vi "Log in MsgList.vi"(8 "error in (no error)":errorcluster, 9 "Username (max 15 characters)":string, 10 "Msg":string, 11 "Function in":refnum<class "Function.lvclass">) -> (0 "error out":errorcluster, 3 "Function out":refnum<class "Function.lvclass">)   [LabVIEW 2016, in "Function Actor.lvlib" / "Function.lvclass"]
uses:
  <userlib>/Common Components/Function Actor/Function.lvclass
  <userlib>/Common Components/Function Actor/Function.lvclass/Function.ctl
  <userlib>/Common Components/Common/Msg MCLstBox Append.vi
  <userlib>/Common Components/Common/Common.lvlib
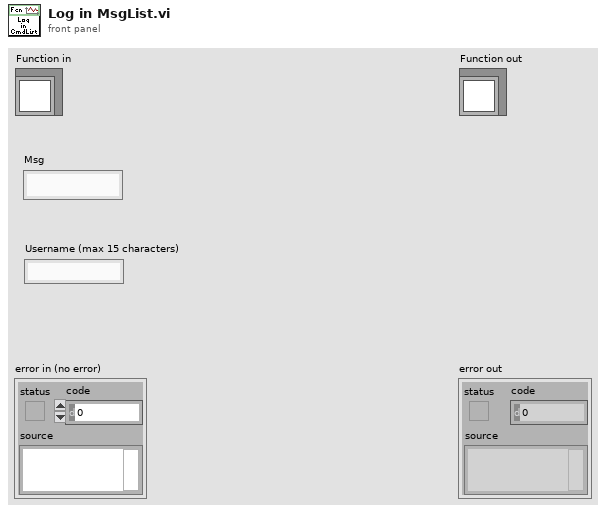
[diagram p1: front panel]
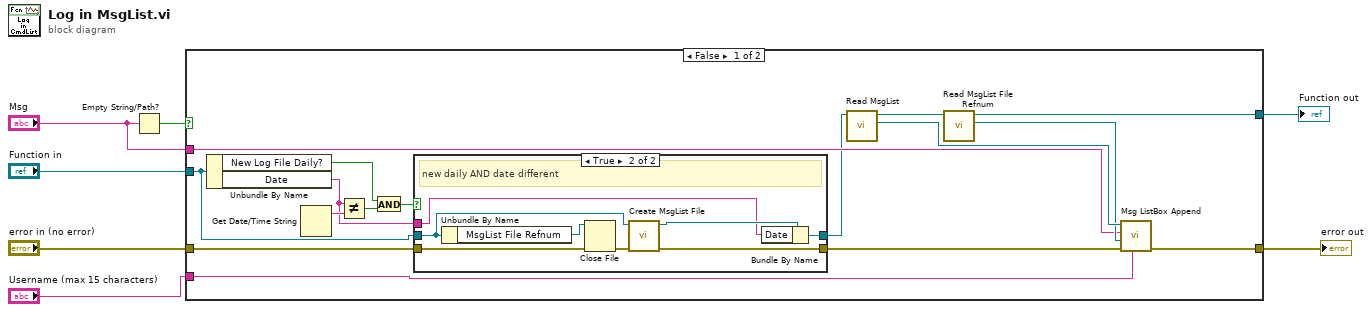
[diagram p0: block diagram]
diagram:
  n1 = Empty String/Path?(string/path="Msg") -> (empty?=w2:bool)
  n2 = case shown="False" w2 {
    tunnel: "Function in" -> [w14 w35]
    tunnel: [w21 w35] -> w6
    tunnel: "error in (no error)" -> [w9 w34]
    tunnel: [w19 w34] -> w4
    tunnel: "Msg" -> [w18 _]
    tunnel: "Username (max 15 characters)" -> [w17 _]
    frame False {
      n3 = Unbundle By Name(w14) -> ("New Log File Daily?"=w11:bool, "Date"=w10:string)
      n4 = Get Date/Time String() -> (date string=w16:string)  [unwired: 3 in, 1 out]
      n5 = Not Equal?(x=w10, y=w16) -> (x != y?=w15:bool)
      n6 = And(x=w11, y=w15) -> (x .and. y?=w12:bool)
      n7 = case shown="True" w12 {
        tunnel: w14 -> [w25 w30]
        tunnel: [w25 w32] -> w13
        tunnel: w10 -> [_ w31]
        tunnel: w9 -> [w24 w27]
        tunnel: [w24 w26] -> w8
        frame False {
        }
        frame True {
          # "new daily AND date different"
          n8 = Unbundle By Name(w30) -> ("MsgList File Refnum"=w29:refnum<file>)
          n9 = Close File(refnum=w29, error in=w27) -> (error out=w28:errorcluster)  [unwired: 1 out]
          n10 = call <userlib>:"Create MsgList File.vi"("error in (no error)"=w28, "Function in"=w30) -> ("error out"=w26:errorcluster, "Function out"=w33:refnum<class "Function.lvclass">)  [unwired: 8 in]
          n11 = Bundle By Name(cluster=w33, "Date"=w31) -> (w32:refnum<class "Function.lvclass">)
        }
      }
      n12 = call <userlib>:"Read MsgList.vi"("Function in"=w13) -> ("Cmd List"=w22:refnum<vi>, "Function out"=w23:refnum<class "Function.lvclass">)  [unwired: 8 in, 1 out]
      n13 = call <userlib>:"Read MsgList File Refnum.vi"("Function in"=w23) -> ("Cmd List File Refnum"=w20:refnum<file>, "Function out"=w21:refnum<class "Function.lvclass">)  [unwired: 8 in, 1 out]
      n14 = call-poly <userlib>:"Msg ListBox Append.vi"("Username (max 15 characters)"=w17, "error in (no error)"=w8, "File Ref"=w20, "Msg"=w18, "MCListbox Refnum"=w22) -> ("error out"=w19:errorcluster)  [unwired: 6 in]
    }
    frame True {
    }
  }
  "error out" <- w4
  "Function out" <- w6
